vi "Scripting_FindCorrespondingSubVITerminal.vi"(0 "SubVITerminalIn":refnum<vi>, 5 "error in":errorcluster) -> (13 "SubVITerminalOutAtSameHeight":refnum<vi>, 14 "SubVITerminalIn Dub":refnum<vi>, 15 "SubVITerminalOut":refnum<vi>[](array[refnum]), 16 "NoTerminalFound":bool, 17 "VI Name":string, 18 "VI Path":path, 19 "error out":errorcluster)   [LabVIEW 2020]
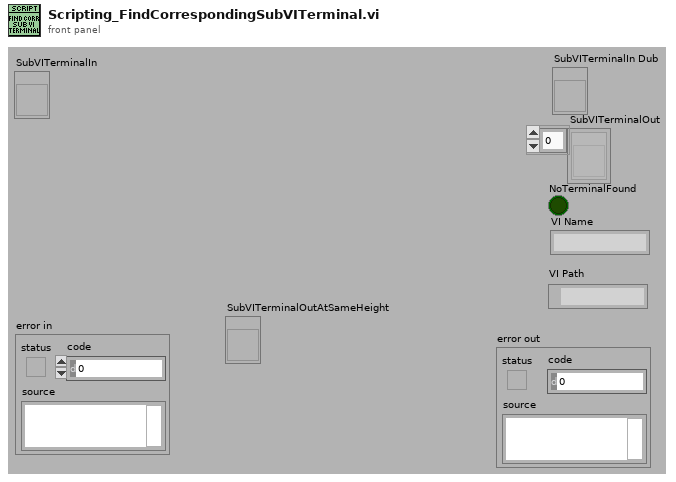
[diagram p1: front panel]
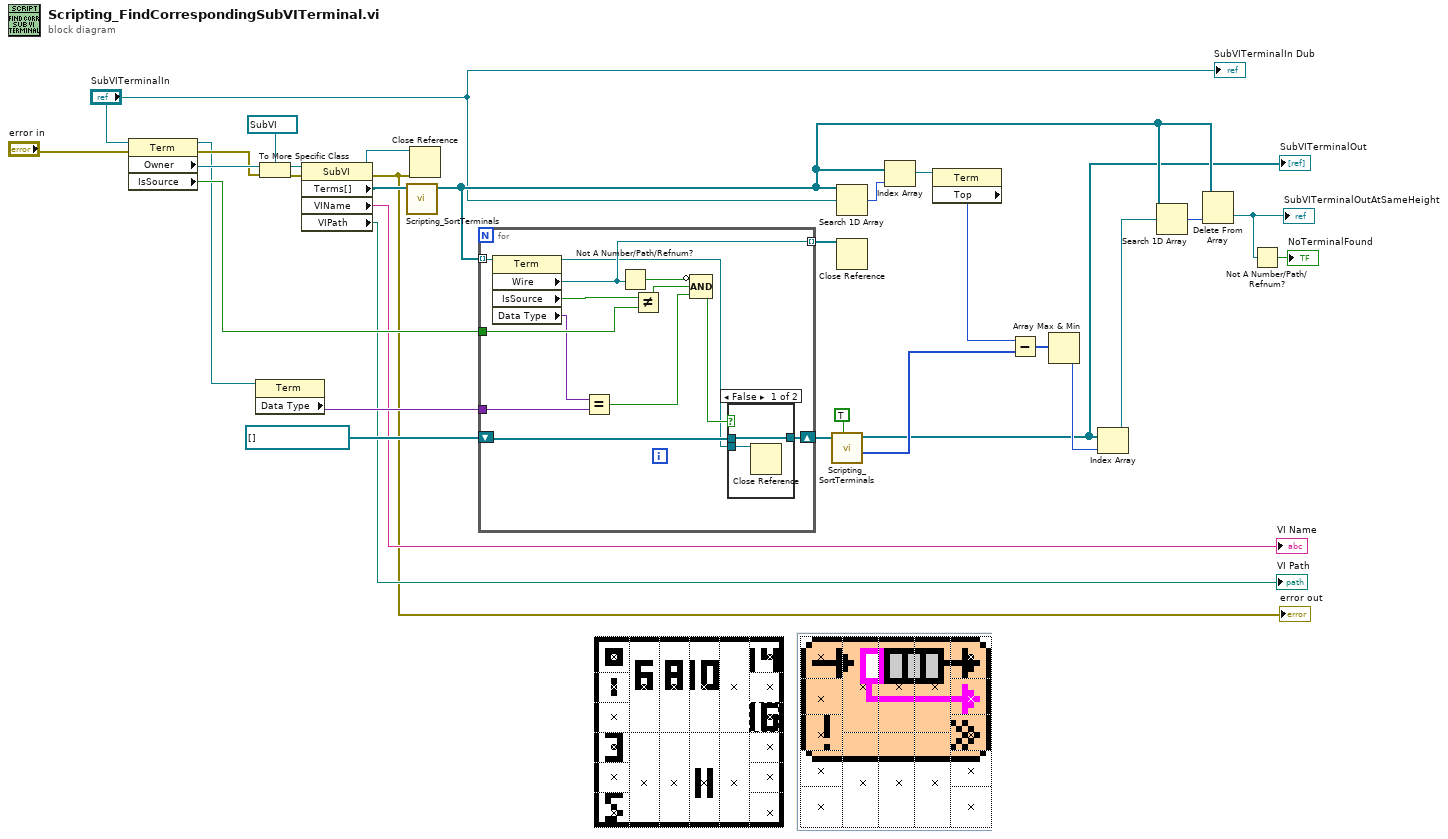
[diagram p0: block diagram]
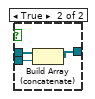
[diagram p2: hidden frame]
diagram:
  n1 = property class="Term"(reference="SubVITerminalIn", error in="error in") -> (reference out=w24:refnum<vi>, error out=w30:errorcluster, "Owner"=w31:refnum<vi>, "IsSource"=w25:bool)
  n2 = property class="Term"(reference=w24) -> ("Data Type"=w23:variant)  [unwired: 1 in, 2 out]
  n3 = To More Specific Class(target class=refnum<vi> refnum ("reference"), reference=w31, error in=w30) -> (specific class reference=w27:refnum<vi>, error out=w9:errorcluster)
  n4 = property class="SubVI"(reference=w27, error in=w9) -> (reference out=w1:refnum<vi>, error out=w2:errorcluster, "Terms[]"=w26:refnum<vi>[], "VIName"=→"VI Name":string, "VIPath"=→"VI Path":path)
  "error out" <- w2
  n5 = call <resource>:"Scripting_SortTerminals.vi"("Terminals[]"=w26) -> ("TerminalsOut[]"=w12:refnum<vi>[])  [unwired: 8 in, 2 out]
  n6 = Close Reference(reference=w1, error in (no error)=w2) -> ()  [unwired: 1 out]
  n7 = for {
    tunnel: w12 -> [w42] mode=indexing
    tunnel: w25 -> [w43]
    tunnel: [w35] -> w21 mode=indexing
    tunnel: w23 -> [w39]
    shift-right: [w34] -> w20
    shift-left: refnum<vi>[] [] -> [w36]
    n8 = property class="Term"(reference=w42) -> (reference out=w32:refnum<vi>, "Wire"=w35:refnum<vi>, "IsSource"=w44:bool, "Data Type"=w38:variant)  [unwired: 1 in, 1 out]
    n9 = Equal?(x=w38, y=w39) -> (x = y?=w37:bool)
    n10 = Not A Number/Path/Refnum?(number/path/refnum=w35) -> (NaN/Path/Refnum?=w41:bool)
    n11 = Not Equal?(x=w44, y=w43) -> (x != y?=w40:bool)
    n12 = Compound Arithmetic op=AND(invert w41, w40, w37) -> (w33:bool)
    n13 = case shown="False" w33 {
      tunnel: w36 -> [w46 w49]
      tunnel: w32 -> [w45 w48]
      tunnel: [w46 w47] -> w34
      frame False {
        n14 = Close Reference(reference=w45) -> ()  [unwired: 1 in, 1 out]
      }
      frame True {
        n15 = Build Array (concatenate)(w49, w48) -> (w47:refnum<vi>[])
      }
    }
  }
  n16 = call <resource>:"Scripting_SortTerminals.vi"("AbsolutPosition(False)"=TRUE, "Terminals[]"=w20) -> ("Ypos"=w16:u32[], "TerminalsOut[]"=w3:refnum<vi>[])  [unwired: 7 in, 1 out]
  "SubVITerminalOut" <- w3
  n17 = Search 1D Array(1D array=w12, element="SubVITerminalIn") -> (index of element=w19:i32)  [unwired: 1 in]
  n18 = Close Reference(reference=w21) -> ()  [unwired: 1 in, 1 out]
  n19 = Index Array(array=w12, index=w19) -> (element=w18:refnum<vi>)
  n20 = property class="Term"(reference=w18) -> ("Top"=w17:i32)  [unwired: 1 in, 2 out]
  n21 = Subtract(x=w17, y=w16) -> (x-y=w15:u32[])
  n22 = Array Max & Min(array=w15) -> (min index (indices)=w14:i32)  [unwired: 3 out]
  n23 = Index Array(array=w3, index=w14) -> (element=w13:refnum<vi>)
  n24 = Search 1D Array(1D array=w12, element=w13) -> (index of element=w11:i32)  [unwired: 1 in]
  n25 = Delete From Array(array=w12, index=w11) -> (deleted portion=w4:refnum<vi>)  [unwired: 1 in, 1 out]
  "SubVITerminalOutAtSameHeight" <- w4
  n26 = Not A Number/Path/Refnum?(number/path/refnum=w4) -> (NaN/Path/Refnum?=→"NoTerminalFound":bool)
  "SubVITerminalIn Dub" <- "SubVITerminalIn"
